vi "Write QoS.vi"(8 "error in (no error)":errorcluster, 10 "QoS":T1, 11 "Subscription in":refnum<class "Subscription.lvclass">) -> (0 "error out":errorcluster, 3 "Subscription out":refnum<class "Subscription.lvclass">)   [LabVIEW 2013, in "MQTT Server.lvlib" / "Subscription.lvclass"]
uses:
  Subscription.lvclass
  Control Packets/ControlPacket/QualityOfService -- enum.ctl
  Subscription.lvclass/Subscription.ctl
  Control Packets/ControlPacket/ControlPacket.lvclass
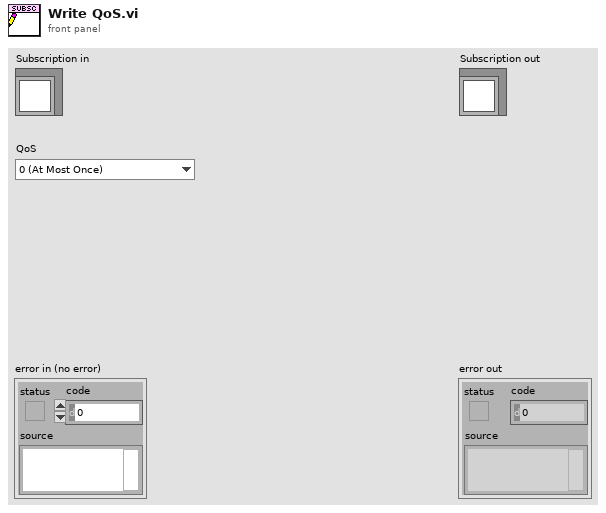
[diagram p1: front panel]
types:
  T1 = typedef "ControlPacket.lvclass/QualityOfService -- enum.ctl" = enum16{"0 (At Most Once)", "1 (At Least Once)", "2 (Exactly Once)"}
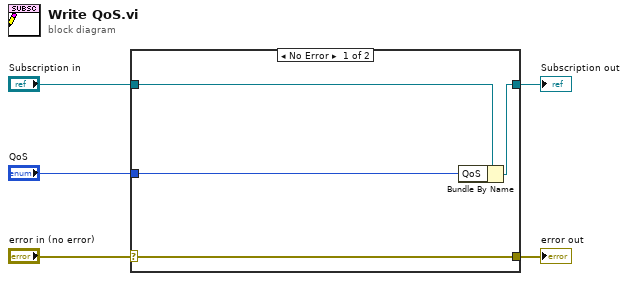
[diagram p0: block diagram]
diagram:
  n1 = case shown="No Error" "error in (no error)" {
    selector: "error in (no error)" -> [w9 w10]
    tunnel: [w9 w10] -> w4
    tunnel: [w7 w11] -> w2
    tunnel: "Subscription in" -> [w8 w11]
    tunnel: "QoS" -> [w6 _]
    frame No Error {
      n2 = Bundle By Name(cluster=w8, "QoS"=w6) -> (w7:refnum<class "Subscription.lvclass">)
    }
    frame Error {
    }
  }
  "error out" <- w4
  "Subscription out" <- w2
